vi "CO Serial CAL & Data Recording & DECADEv3.3.vi"() -> ()   [LabVIEW 2014]
uses:
  <vilib>/Platform/TimedLoop/XDataNode/timing_clust.ctl
  <vilib>/Platform/TimedLoop/XDataNode/nitl_modes.ctl
  <vilib>/Platform/TimedLoop/XDataNode/wakeup.ctl
  C:/Program Files (x86)/National Instruments/LabVIEW 2014/examples/Data Communication/Network Streams/Simple Network Streams/support/Network Stream Command.ctl
  <vilib>/Utility/error.llb/whitespace.ctl
  <vilib>/Instr/_visa.llb/VISA Configure Serial Port (Instr).vi
  <vilib>/Utility/tcp.llb/UDP Multicast Write-Only Open.vi
  <vilib>/platform/TimedLoop/XDataNode/XDataNode.xnode
  <vilib>/Platform/TimedLoop/XDataNode/XDNodeRunTimeDep.lvlib
panel:
  out "Stop File Write":bool
  out "Default file name":string
  in  "Flight Number 2":string="XXXX"
  out "status":bool
  out "CO Vacuum":bool
  out "CO CAL":bool
  out "error out":errorcluster
  out "CO Vacuum?":i16
  out "Control data":i32[](array[numeric])
  out "Control data out":string
  in  "VISA resource name":refnum<visa-resource-name>="ASRL8::INSTR"
  out "Serial VISA error":errorcluster
  out "SEPTIC TCP Error Out":errorcluster
  out "TCP packet\nSend To SEPTIC":bool
  in  "msec to wait":u32=330 caption="mSec to Wait"
  out "UDP Time Stamp Offset":i32=1
  out "Scan from String Error \nCounter from process loop":i32
  out "TCP Binary Packet":string
  in  "ue9LJ temp":u16
  out "FISH TCP Error Out":errorcluster
  out "TCP packet\nSend To FISH":bool
  out "UDP_Out_Error Out":errorcluster
  out "Data Array":string[](array[string])
  out "UDP_Out Status":bool
  out "Data Process Status":bool
  out "Command In":string[](array[string])
  out "ERR Counter":i32
  out "UDP_Out":string
  out "UDP_Pack_num":u32
  out "Flight Number":string
  out "OK RAW COUNTER":i32
  out "IN_CAL?":bool
  out "Redundent DATA":string
  out "Data String":string
  out "CO_Data_Buffer":string[](array[string])
  out "RAW DATA":string
  out "loop count":i32
  out "Number of Read error":i32
  out "Command In":string
  # "Pre-flight"
  # "CONC"
  # "SIG"
  # "SENS"
  # "ZERO"
  # "Lamp flow controller"
  # "Lamp temperature"
  # "Monochromater flow controller"
  # "Monochromater temperature"
  # "Monochromater pressure"
  # "Fluorescence cell pressure"
  # "Calibration gas pressure"
  # "Cell temperature"
  # "Calibration Concentration"
  # "ERROR number"
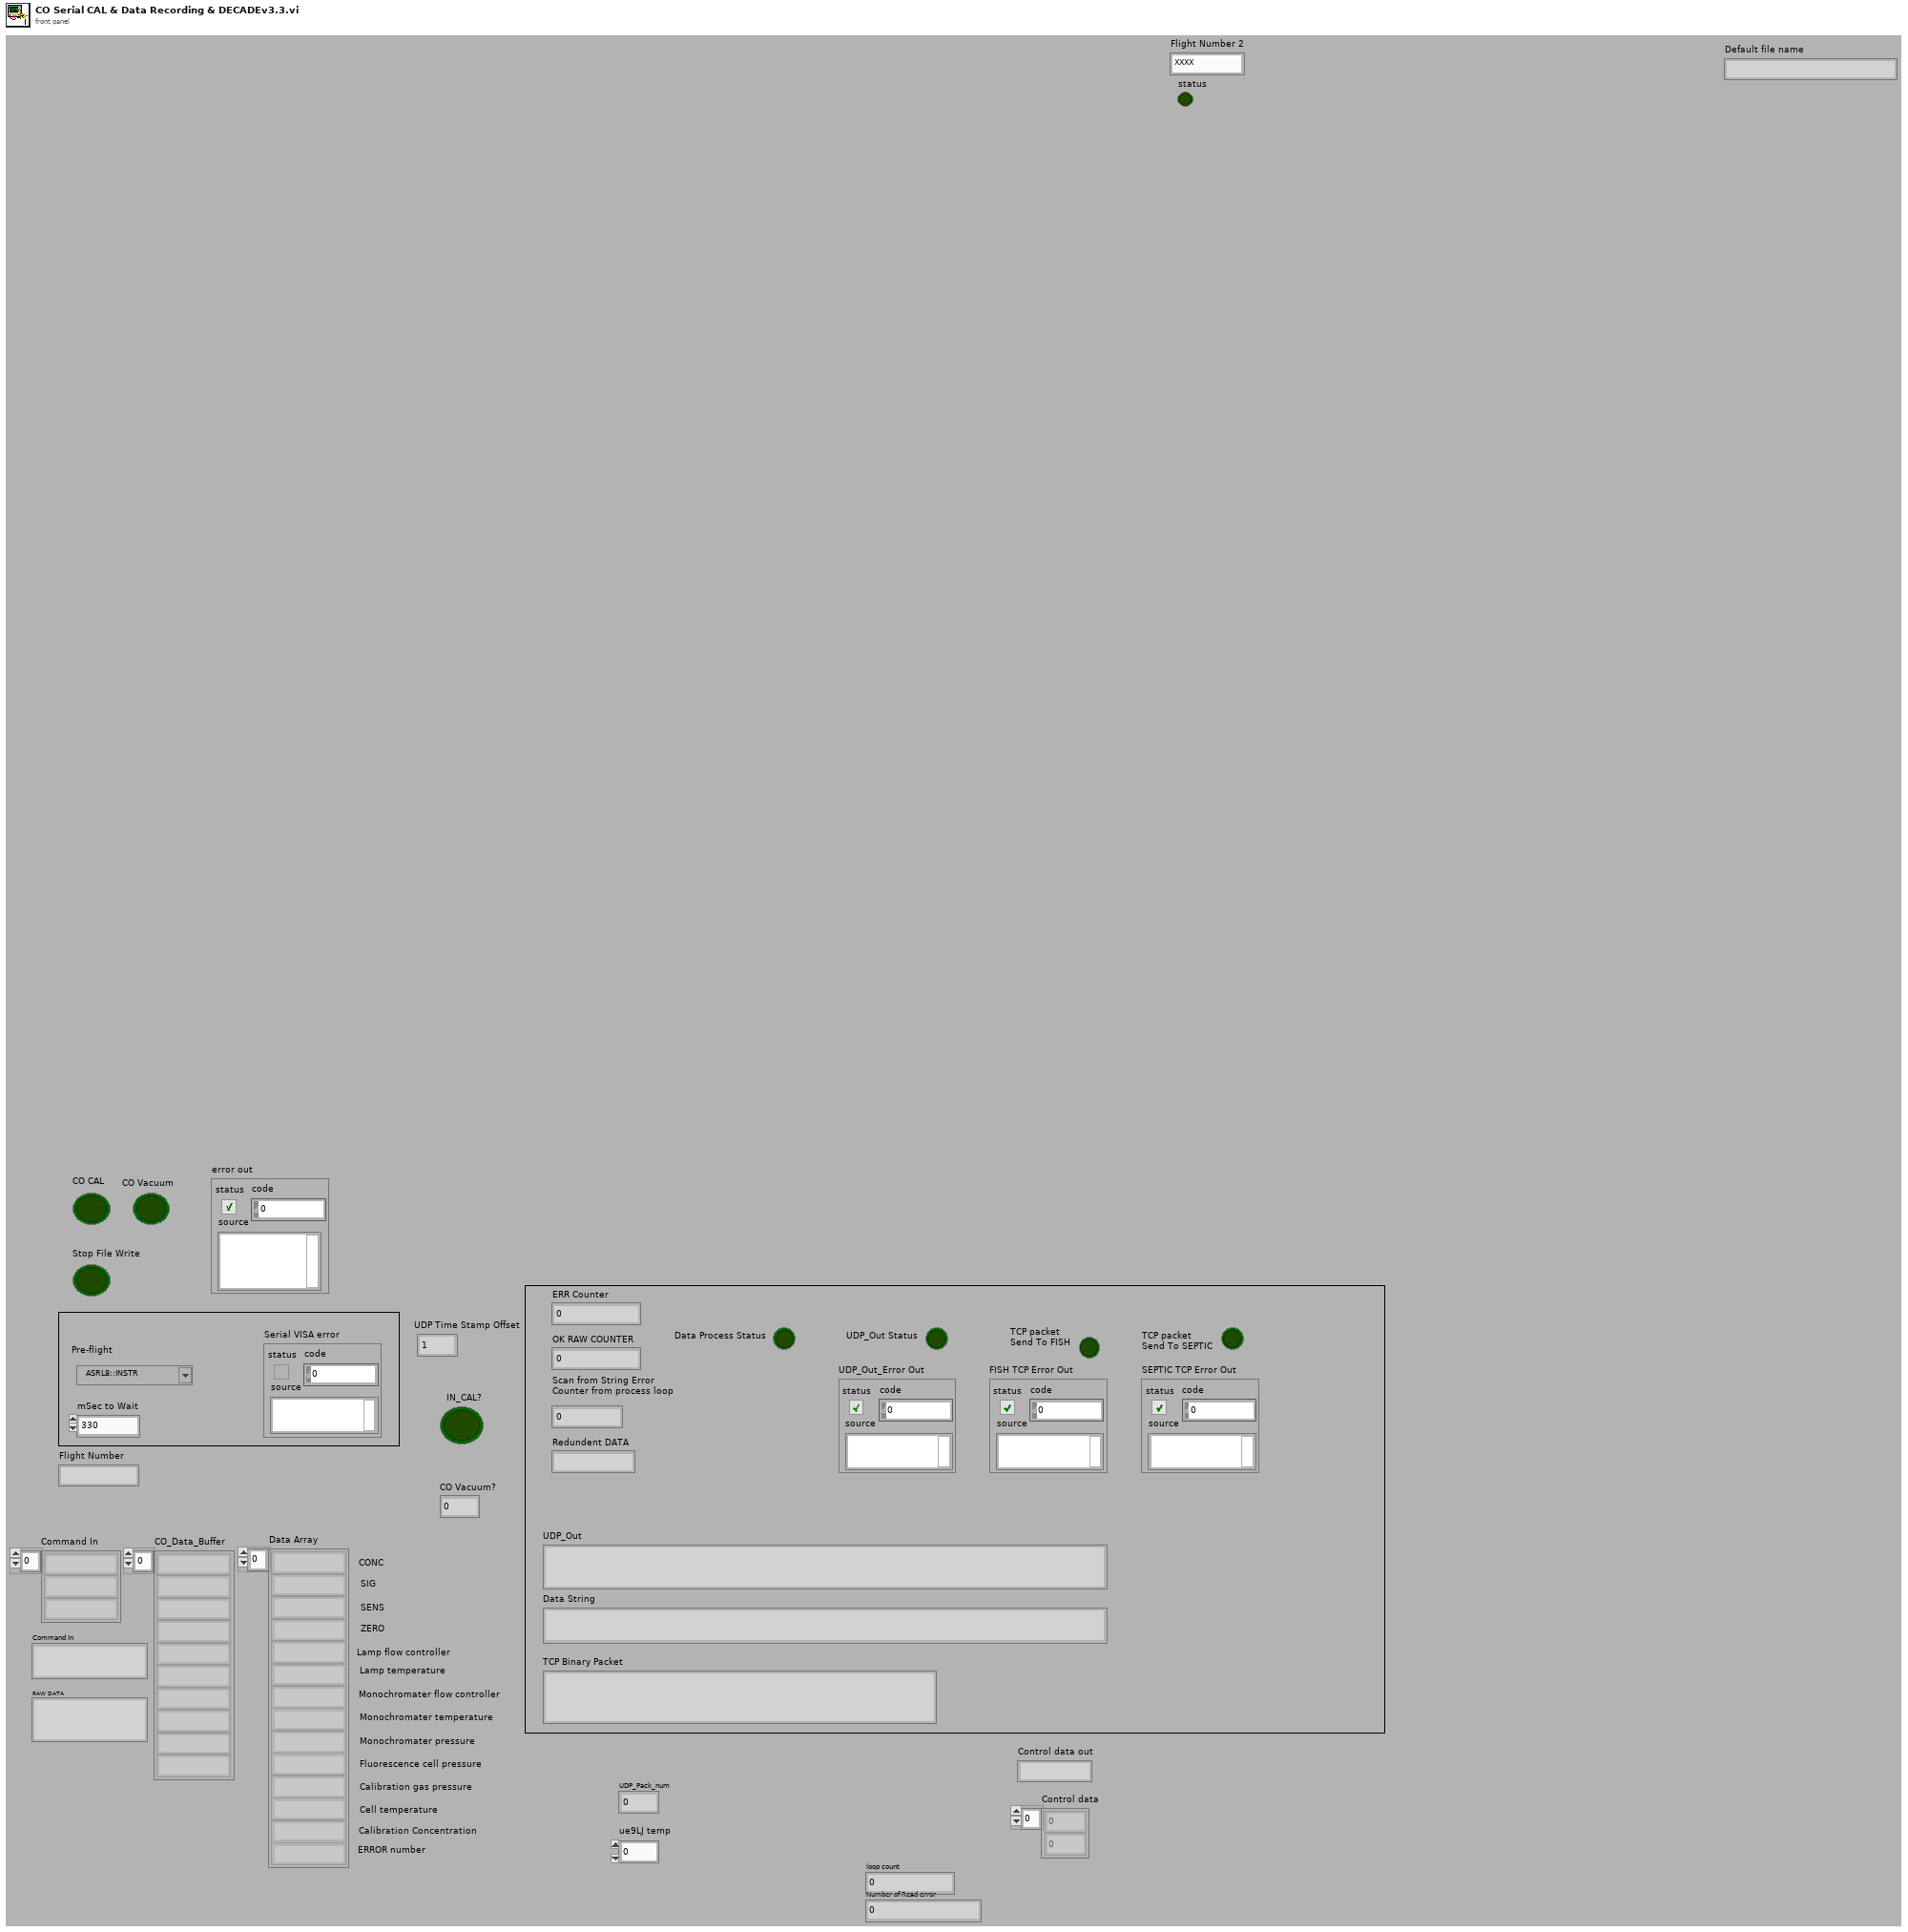
[diagram p1: front panel]
types:
  T1 = typedef "XDNodeRunTimeDep.lvlib/timing_clust.ctl" = cluster{"Expected End [f-1]":u64, "Actual End [f-1]":u64, "Finished Late? [f-1]":bool, "Expected End [i-1]":u64, "Actual End [i-1]":u64, "Finished Late? [i-1]":bool, "Expected Start [i]":u64, "Actual Start [i]":u64, "Expected Start [f]":u64, "Actual Start [f]":u64, "Source Name":string, "Structure Name":string, "Period":i64, "Deadline":i64, "Offset":i64, "Start":i64, "Priority":i32, "Timeout":i32, "Mode":T2, "Wakeup Reason":T3, "Error":errorcluster, "Source Type":string, "Secondary Source Type":string, "Global End Time":u64, "Global Start Time":u64, "Frame Duration":u64, "Iteration Duration":u64, "Assigned CPU":i32, "I/O Scan Engine Mode":u32}
  T2 = typedef "XDNodeRunTimeDep.lvlib/nitl_modes.ctl" = enum32{"No Change", "Process missed periods, maintain original phase", "Discard missed periods, maintain original phase", "Process missed periods, ignore original phase", "Discard missed periods, ignore original phase"}
  T3 = typedef "XDNodeRunTimeDep.lvlib/wakeup.ctl" = enum32{"Normal", "Aborted", "Asynchronous wakeup", "Timing source error", "Timed loop error", "Timeout"}
  T4 = typedef "Network Stream Command.ctl" = cluster{"Message":string, "Message Data":variant}
  T5 = enum16{"open", "replace", "create", "open or create", "replace or create", "replace or create with confirmation"}
  T6 = typedef "whitespace.ctl" = u16
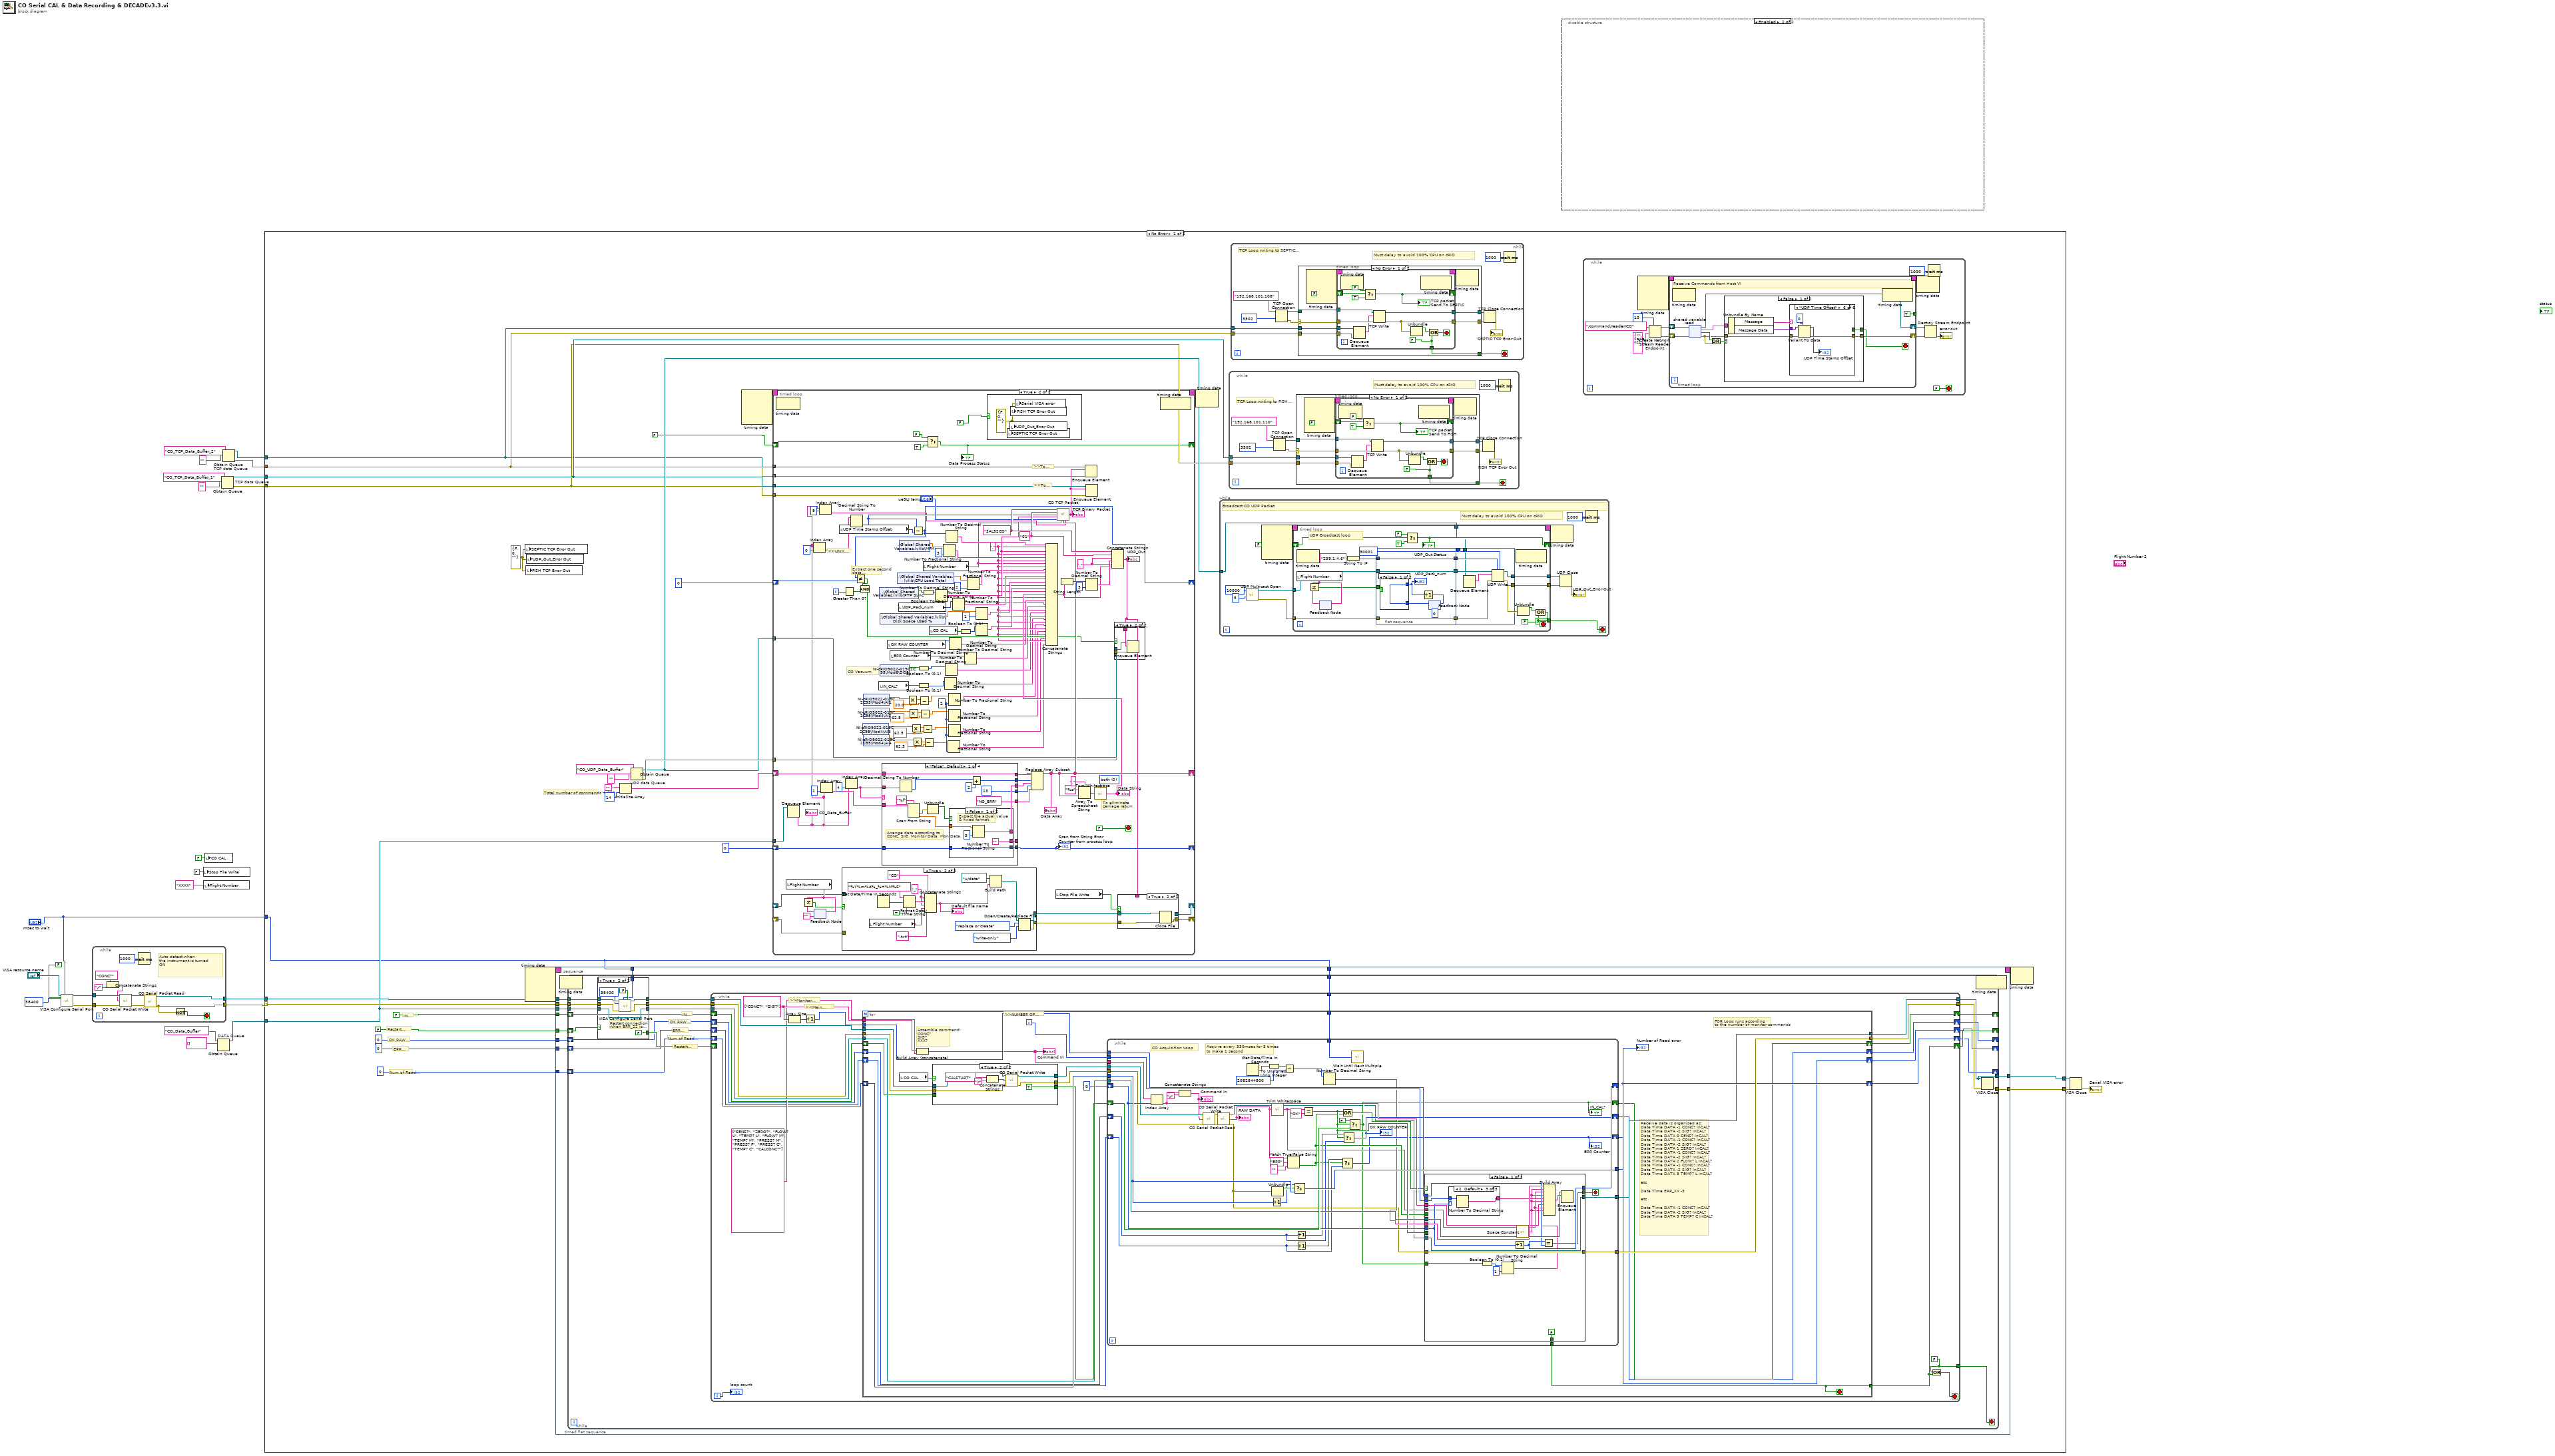
[diagram p0: block diagram]
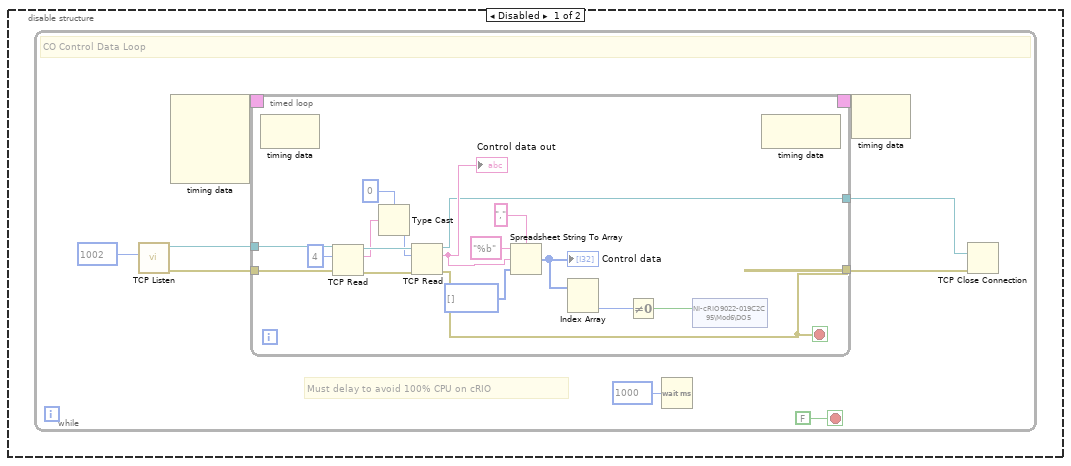
[diagram p2: hidden frame]
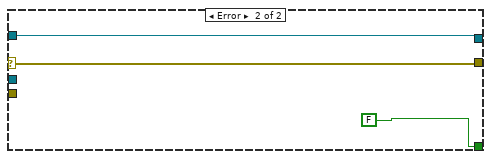
[diagram p3: hidden frame]
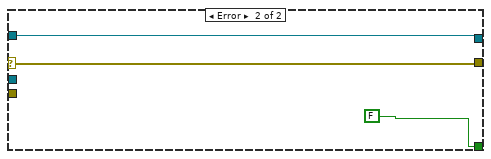
[diagram p4: hidden frame]
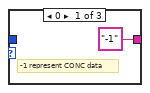
[diagram p6: hidden frame]
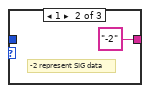
[diagram p7: hidden frame]
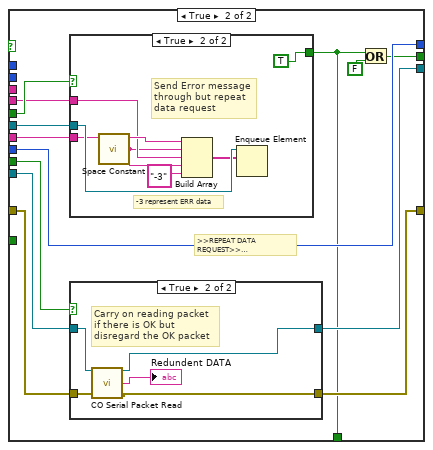
[diagram p8: hidden frame]
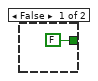
[diagram p10: hidden frame]
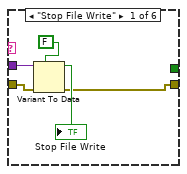
[diagram p12: hidden frame]
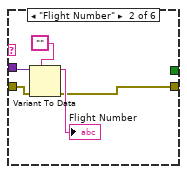
[diagram p13: hidden frame]
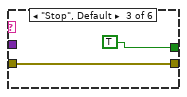
[diagram p14: hidden frame]
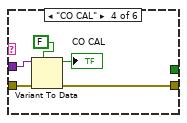
[diagram p15: hidden frame]
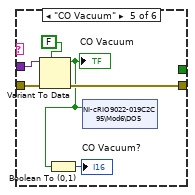
[diagram p16: hidden frame]
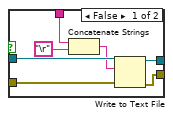
[diagram p19: hidden frame]
diagram:
  n1 = call-poly "VISA Configure Serial Port"("VISA resource name"="VISA resource name", "timeout (10sec)"="msec to wait", "Enable Termination\nChar (T)"=FALSE ("Enable Termination\nChar (T)"), "baud rate (9600)"=u32 38400) -> ("VISA resource name out"=w12:refnum<visa-resource-name>, "error out"=w11:errorcluster)  [unwired: 10 in]
  n2 = while {
    tunnel: w12 -> [w36]
    tunnel: w11 -> [w35]
    tunnel: [w29] -> w10
    tunnel: [w30] -> w9
    stop <- w34 stop-if-true
    # "Auto detect when\nthe instrument is turned \nON"
    n3 = Concatenate Strings("CONC?" ("Data in"), "\r") -> (w26:string)
    n4 = call "CO Serial Packet Write.vi"("VISA resource name In"=w36, "Data in"=w26, "error in (no error)"=w35) -> ("VISA resource name Out"=w32:refnum<visa-resource-name>, "error out"=w31:errorcluster)  [unwired: 11 in]
    n5 = Wait (ms)(milliseconds to wait=u32 1000) -> ()  [unwired: 1 out]
    n6 = call "CO Serial Packet Read.vi"("VISA resource In"=w32, "error in"=w31) -> ("VISA resource Out"=w29:refnum<visa-resource-name>, "error out"=w30:errorcluster)  [unwired: 11 in, 1 out]
    n7 = Not(x=w30) -> (.not. x?=w34:bool)
  }
  n8 = local write "Stop File Write"(FALSE ("Stop File Write")) -> ()
  n9 = local write "Flight Number"("XXXX" ("Flight Number")) -> ()
  n10 = local write "CO CAL"(FALSE ("CO CAL")) -> ()
  n11 = Obtain Queue "DATA Queue"(name (unnamed)="CO_Data_Buffer", element data type=string[] []) -> (queue out=w23:refnum<queue>)  [unwired: 3 in, 2 out]
  n12 = Obtain Queue "TCP data Queue"(name (unnamed)="CO_TCP_Data_Buffer_1", element data type="") -> (queue out=w22:refnum<queue>, error out=w21:errorcluster)  [unwired: 3 in, 1 out]
  n13 = Obtain Queue "TCP data Queue"(name (unnamed)="CO_TCP_Data_Buffer_2", element data type="") -> (queue out=w20:refnum<queue>, error out=w19:errorcluster)  [unwired: 3 in, 1 out]
  n14 = case shown="No Error" w9 {
    selector: w9 -> [w64 w714]
    tunnel: w10 -> [w65 w713]
    tunnel: [w66 w714] -> w15
    tunnel: [w42 w713] -> w14
    tunnel: w23 -> [w63 _]
    tunnel: w22 -> [w52 _]
    tunnel: w21 -> [w51 _]
    tunnel: w20 -> [w50 _]
    tunnel: w19 -> [w49 _]
    tunnel: "msec to wait" -> [w37 _]
    frame No Error {
      w48 = errorcluster {"status"=FALSE, "code"=0, "source"=""} ("UDP_Out_Error Out")
      # "Restart connection?"
      # "IN CAL?"
      # "OK RAW Counter"
      # "ERR Counter"
      # "Num of Read Error"
      # "Total number of commands + ERR"
      n15 = node-c288() -> (w39:T1)  [unwired: 4 in]
      n16 = local write "SEPTIC TCP Error Out"(w48) -> ()
      n17 = local write "FISH TCP Error Out"(w48) -> ()
      n18 = local write "UDP_Out_Error Out"(w48) -> ()
      n19 = timed-sequence {
        timing: w39 -> [_]
        timing-out: [_] -> w38
        tunnel: [w162] -> w66
        tunnel: w65 -> [w161]
        tunnel: w64 -> [w160]
        tunnel: w63 -> [w159]
        tunnel: FALSE -> [w158]
        tunnel: 0 -> [w157]
        tunnel: 0 -> [w156]
        tunnel: 0 -> [w155]
        tunnel: FALSE ("IN_CAL?") -> [w154]
        tunnel: [w153] -> w42
        tunnel: w37 -> [w152]
        tunnel: w37 -> [w151]
        n20 = timed-flat-sequence {
          tunnel: [w174] -> w162
          tunnel: w161 -> [w173]
          tunnel: w160 -> [w172]
          tunnel: w159 -> [w171]
          tunnel: w158 -> [w170]
          tunnel: w157 -> [w169]
          tunnel: w156 -> [w168]
          tunnel: w155 -> [w167]
          tunnel: w154 -> [w166]
          tunnel: [w165] -> w153
          tunnel: w152 -> [w164]
          tunnel: w151 -> [w163]
          n21 = node-c288() -> ()  [unwired: 1 in, 1 out]
          n22 = while {
            tunnel: [w179] -> w174
            tunnel: w173 -> [w196]
            tunnel: w172 -> [w195]
            tunnel: w171 -> [w193]
            shift-right: [w190] -> _
            shift-left: w170 -> [w191]
            shift-right: [w186] -> _
            shift-left: w169 -> [w187]
            shift-right: [w183] -> _
            shift-left: w168 -> [w185]
            shift-right: [w182] -> _
            shift-left: w167 -> [w184]
            shift-right: [w180] -> _
            shift-left: w166 -> [w181]
            tunnel: [w177] -> w165
            tunnel: w164 -> [w176]
            tunnel: w163 -> [w175]
            stop <- w189 stop-if-true
            # "Restart connection?"
            # "Num of Read Error"
            # "ERR Counter"
            # "IN CAL?"
            # "OK RAW Counter"
            n23 = case shown="True" w191 {
              selector: w191 -> [w198 _]
              tunnel: [w201 w207] -> w197
              tunnel: w196 -> [w201 w208]
              tunnel: [w200 w206] -> w194
              tunnel: w195 -> [w200 w205]
              tunnel: [w199 w210] -> w192
              tunnel: w193 -> [w199 w210]
              tunnel: [w198 FALSE] -> w188
              tunnel: w175 -> [_ w202]
              frame False {
              }
              frame True {
                # "Restart connection\nwhen ERR_22 is detected"
                n24 = call-poly "VISA Configure Serial Port"("VISA resource name"=w208, "timeout (10sec)"=w202, "Enable Termination\nChar (T)"=FALSE ("Enable Termination\nChar (T)"), "baud rate (9600)"=u32 38400, "error in (no error)"=w205) -> ("VISA resource name out"=w207:refnum<visa-resource-name>, "error out"=w206:errorcluster)  [unwired: 9 in]
              }
            }
            n25 = while {
              tunnel: [w232] -> w178
              tunnel: w197 -> [w231]
              tunnel: w194 -> [w230]
              tunnel: [w229] -> w177
              tunnel: w192 -> [w228]
              shift-right: [w219] -> w186
              shift-left: w187 -> [w223]
              shift-right: [w218] -> w183
              shift-left: w185 -> [w222]
              shift-right: [w217] -> w180
              shift-left: w181 -> [w221]
              shift-right: [w216] -> w182
              shift-left: w184 -> [w220]
              tunnel: [w212] -> w189
              shift-right: [w213] -> w190
              shift-left: w188 -> [_]
              tunnel: w176 -> [w211]
              i -> [w215]
              stop <- w214 stop-if-true
              w212 = FALSE
              w227 = string[] ["CONC?", "SIG?"]
              # ">>Main commands>>"
              # ">>Monitor Command>>"
              n26 = Array Size(array=w227) -> (size(s)=w224:i32)
              n27 = Increment(x=w224) -> (x+1=w226:i32)
              n28 = for {
                tunnel: w231 -> [w252]
                tunnel: w230 -> [w251]
                tunnel: [w257] -> w232
                shift-right: [w255] -> w216
                shift-left: w220 -> [w256]
                tunnel: [w254] -> w229
                tunnel: w228 -> [w253]
                tunnel: w226 -> [w247]
                shift-right: [w245] -> w217
                shift-left: w221 -> [w246]
                shift-right: [w243] -> w218
                shift-left: w222 -> [w244]
                shift-right: [w241] -> w219
                shift-left: w223 -> [w242]
                tunnel: string[] ["SENS?", "ZERO?", "FLOW? L", "TEMP? L", "FLOW? M", "TEMP? M", "PRESS? M", "PRESS? F", "PRESS? C", "TEMP? C", "CALCONC?"] -> [w238] mode=indexing
                tunnel: w227 -> [w239]
                tunnel: [w236] -> w213
                tunnel: w211 -> [w234]
                i -> [w237]
                stop <- w236 stop-if-true
                # "Receive data is organised as:\nDate Time DATA -1 CONC? InCAL?\nDate Time DATA -2 SIG? InCAL?\nDate Time DATA 0 SENS? InCAL?\nDate Time DATA -1 CONC? InCAL?\nDate Time DATA -2 SIG? InCAL?\nDate Time DATA 1 ZERO? InCAL?\nDate Time DATA -1 CONC? InCAL?\nDate Time DATA -2 SIG? InCAL?\nDate Time DATA 2 FLOW? L InCAL?\nDate Time DATA -1 CONC? InCAL?\nDate Time DATA -2 SIG? InCAL?\nDate Time DATA 3 TEMP? L InCAL?\n\netc\n\nDate Time ERR_XX -3\n\netc\n\nDate Time DATA -1 CONC? InCAL?\nDate Time DATA -2 SIG? InCAL?\nDate Time DATA 9 TEMP? C InCAL?"
                # "FOR Loop runs according\nto the number of monitor commands"
                # "Assemble command:\nCONC?\nSIG?\nXXX?"
                # ">>NUMBER OF COMMANDS>>"
                n29 = local read "CO CAL"() -> (w233:bool)
                n30 = Build Array (concatenate)(w239, w238) -> (w240:string[])
                "Command In" <- w240
                n31 = case shown="True" w233 {
                  tunnel: w252 -> [w357 w359]
                  tunnel: w251 -> [w356 w362]
                  tunnel: [w357 w360] -> w250
                  tunnel: [w356 w361] -> w249
                  tunnel: [w355 TRUE ("IN_CAL?")] -> w248
                  tunnel: w246 -> [w355 _]
                  frame False {
                  }
                  frame True {
                    n32 = Concatenate Strings("CALSTART" ("string"), "\r") -> (w358:string)
                    n33 = call "CO Serial Packet Write.vi"("VISA resource name In"=w359, "Data in"=w358, "error in (no error)"=w362) -> ("VISA resource name Out"=w360:refnum<visa-resource-name>, "error out"=w361:errorcluster)  [unwired: 11 in]
                  }
                }
                n34 = while {
                  tunnel: w249 -> [w264]
                  tunnel: [w291] -> w257
                  tunnel: w256 -> [w303]
                  tunnel: [w302] -> w255
                  tunnel: w240 -> [w295]
                  tunnel: [w292] -> w254
                  tunnel: w253 -> [w290]
                  tunnel: w250 -> [w266]
                  shift-right: [w267] -> w245
                  shift-left: w248 -> [w297]
                  shift-right: [w294] -> _
                  shift-left: 0 -> [w296]
                  tunnel: w247 -> [w287]
                  shift-right: [w284] -> w243
                  shift-left: w244 -> [w285]
                  shift-right: [w278] -> w241
                  shift-left: w242 -> [w280]
                  tunnel: w237 -> [w277]
                  tunnel: [w272] -> w236
                  tunnel: w234 -> [w258]
                  stop <- w293 stop-if-true
                  # "Acquire every 330msec for 3 times\nto make 1 second"
                  # "CO Acquisition Loop"
                  n35 = Index Array(array=w295, index=w296) -> (element=w289:string)
                  n36 = Concatenate Strings(w289, "\r") -> (w265:string)
                  "Command In" <- w265
                  n37 = call "CO Serial Packet Write.vi"("VISA resource name In"=w266, "Data in"=w265, "error in (no error)"=w264) -> ("VISA resource name Out"=w262:refnum<visa-resource-name>, "error out"=w263:errorcluster)  [unwired: 11 in]
                  n38 = call "CO Serial Packet Read.vi"("VISA resource In"=w262, "error in"=w263) -> ("VISA resource Out"=w261:refnum<visa-resource-name>, "Data Out"=w259:string, "error out"=w260:errorcluster)  [unwired: 11 in]
                  "RAW DATA" <- w259
                  n39 = Get Date/Time In Seconds() -> (seconds since 1Jan1904=w273:timestamp)
                  n40 = To Unsigned Long Integer(number=w273) -> (unsigned 32bit integer=w276:u32)
                  n41 = Increment(x=w303) -> (x+1=w299:i32)
                  n42 = call <vilib>:"Trim Whitespace.vi"("string"=w259) -> ("trimmed string"=w271:string)  [unwired: 1 in]
                  n43 = Unbundle(w260) -> ("status"=w300:bool)  [unwired: 2 out]
                  n44 = Subtract(x=w276, y=u32 2082844800) -> (x-y=w268:u32)
                  n45 = Match True/False String(2:"" ("false string"), 3:"ERR" ("true string"), 4:w259) -> (0:w279:bool)  [unwired: 1 out]
                  n46 = Select(t=w299, s=w300, f=w303) -> (s? t:f=w302:i32)
                  n47 = Increment(x=w285) -> (x+1=w286:i32)
                  n48 = Increment(x=w280) -> (x+1=w281:i32)
                  n49 = Equal?(x=w271, y="OK" ("string")) -> (x = y?=w282:bool)
                  n50 = Number To Decimal String(number=w268) -> (decimal integer string=w274:string)  [unwired: 1 in]
                  n51 = Select(t=w281, s=w279, f=w280) -> (s? t:f=w278:i32)
                  "ERR Counter" <- w278
                  n52 = Select(t=w286, s=w282, f=w285) -> (s? t:f=w284:i32)
                  "OK RAW COUNTER" <- w284
                  n53 = Compound Arithmetic op=OR(w282, w279) -> (w283:bool)
                  n54 = Select(t=FALSE, s=w282, f=w297) -> (s? t:f=w267:bool)
                  "IN_CAL?" <- w267
                  n55 = call "Wait Until Next Multiple"("Count(mSec)"=w258) -> ()  [unwired: 1 out]
                  n56 = case shown="False" w283 {
                    tunnel: w296 -> [w311 w339]
                    tunnel: [w322 w339] -> w294
                    tunnel: [w316 w329] -> w293
                    tunnel: w261 -> [w321 w338]
                    tunnel: w260 -> [w320 w337]
                    tunnel: [w321 w336] -> w292
                    tunnel: [w320 w335] -> w291
                    tunnel: w290 -> [w318 w333]
                    tunnel: w271 -> [w309 w331]
                    tunnel: w289 -> [w312 _]
                    tunnel: w274 -> [w317 w332]
                    tunnel: w279 -> [_ w334]
                    tunnel: w287 -> [w315 _]
                    tunnel: w282 -> [_ w330]
                    tunnel: w277 -> [w314 _]
                    tunnel: [FALSE w327] -> w272
                    tunnel: w267 -> [w308 _]
                    frame False {
                      n57 = case shown="2, Default" w311 {
                        tunnel: w314 -> [_ _ w326]
                        tunnel: ["-1" "-2" w325] -> w313
                        frame 0 {
                          # "-1 represent CONC data"
                        }
                        frame 1 {
                          # "-2 represent SIG data"
                        }
                        frame 2, Default {
                          n58 = Number To Decimal String(number=w326) -> (decimal integer string=w325:string)  [unwired: 1 in]
                        }
                      }
                      n59 = Boolean To (0,1)(Boolean=w308) -> (0, 1=w307:i16)
                      n60 = Number To Decimal String(number=w307, width (-)=i16 1) -> (decimal integer string=w304:string)
                      n61 = Increment(x=w311) -> (x+1=w322:i32)
                      n62 = call <vilib>:"Space Constant.vi"() -> ("String"=w305:string)
                      n63 = Equal?(x=w322, y=w315) -> (x = y?=w316:bool)
                      n64 = Build Array(w317, w305, w309, w305, w313, w305, w312, w309, w305, w304) -> (w319:string[])
                      n65 = Enqueue Element(queue=w318, element=w319) -> ()  [unwired: 2 in, 3 out]
                    }
                    frame True {
                      # ">>REPEAT DATA REQUEST>>\nif OK or ERR"
                      n66 = case shown="True" w334 {
                        tunnel: w333 -> [_ w354]
                        tunnel: w332 -> [_ w352]
                        tunnel: w331 -> [_ w351]
                        tunnel: [FALSE TRUE] -> w327
                        frame False {
                        }
                        frame True {
                          # "-3 represent ERR data"
                          # "Send Error message\nthrough but repeat\ndata request"
                          n67 = call <vilib>:"Space Constant.vi"() -> ("String"=w350:string)
                          n68 = Build Array(w352, w350, w351, w350, "-3" ("element")) -> (w353:string[])
                          n69 = Enqueue Element(queue=w354, element=w353) -> ()  [unwired: 2 in, 3 out]
                        }
                      }
                      n70 = case shown="True" w330 {
                        tunnel: w338 -> [w340 w345]
                        tunnel: w337 -> [w341 w346]
                        tunnel: [w340 w344] -> w336
                        tunnel: [w341 w342] -> w335
                        frame False {
                        }
                        frame True {
                          # "Carry on reading packet\nif there is OK but\ndisregard the OK packet"
                          n71 = call "CO Serial Packet Read.vi"("VISA resource In"=w345, "error in"=w346) -> ("VISA resource Out"=w344:refnum<visa-resource-name>, "Data Out"=→"Redundent DATA":string, "error out"=w342:errorcluster)  [unwired: 11 in]
                        }
                      }
                      n72 = Or(x=w327, y=FALSE) -> (x .or. y?=w329:bool)
                    }
                  }
                }
                "Number of Read error" <- w255
              }
              n73 = Or(x=w212, y=w213) -> (x .or. y?=w214:bool)
              "loop count" <- w215
            }
            n74 = VISA Close(VISA resource name=w177, error in (no error)=w178) -> (error out=w179:errorcluster)
          }
          n75 = node-c288() -> ()  [unwired: 1 in, 1 out]
        }
      }
      n76 = Initialize Array("", 14) -> (w60:string[])
      n77 = Obtain Queue "UDP data Queue"(name (unnamed)="CO_UDP_Data_Buffer", element data type="") -> (queue out=w55:refnum<queue>, error out=w56:errorcluster)  [unwired: 3 in, 1 out]
      n78 = node-c288() -> (w41:T1)  [unwired: 4 in]
      n79 = timed-loop {
        tunnel: w63 -> [w547]
        shift-right: [w518] -> _
        shift-left: w60 -> [w535]
        shift-right: [w522] -> _
        shift-left: FALSE -> [w525]
        tunnel: w52 -> [w517]
        tunnel: w51 -> [w516]
        tunnel: w55 -> [w514]
        tunnel: w56 -> [w513]
        shift-right: [w511] -> _
        shift-left: 0 -> [w512]
        shift-right: [w498] -> _
        shift-left: 0 -> [w505]
        tunnel: w50 -> [w503]
        tunnel: w49 -> [w502]
        timing: w41 -> [_]
        timing-out: [_] -> w40
        shift-right: [w487] -> _
        shift-left: _ -> [w480]
        shift-right: [w478] -> _
        shift-left: _ -> [w479]
        i -> [w508]
        stop <- FALSE stop-if-true
        w461 = 62.5 ("y")
        w462 = 62.5 ("y")
        w465 = 62.5 ("y")
        w468 = 20.0 ("y")
        w491 = i16 2 ("precision (6)")
        w527 = T6 0 items=["both", "start of string", "end of string"] ("location (both)")
        w443 = ","
        w520 = "01"
        w538 = ","
        w521 = "$AL52CO"
        # "CO Vacuum"
        # ">>To SEPTIC>>"
        # ">>To FISH>>"
        # "Extract one second data\nfor UDP sending"
        # ">>UNIX TIME>>"
        # "To eliminate\ncarriage return"
        n80 = node-c288() -> ()  [unwired: 1 in, 1 out]
        n81 = local read "Flight Number"() -> (w485:string)
        n82 = Dequeue Element(queue=w547) -> (element=w494:string[])  [unwired: 2 in, 3 out]
        "CO_Data_Buffer" <- w494
        n83 = Index Array(array=w494, index=0) -> (element=w506:string)
        n84 = feedback #1("" ("Flight Number")) -> (w484:string)
        n85 = Not Equal?(x=w485, y=w484) -> (x != y?=w483:bool)
        n86 = feedback-in #1(w485) -> ()
        n87 = Index Array(array=w494, index=9) -> (element=w493:string)
        n88 = Index Array(array=w494, index=2) -> (element=w533:string)
        n89 = local read "UDP Time Stamp Offset"() -> (w432:i32)
        n90 = case shown="True" w483 {
          tunnel: [w549 w551] -> w482
          tunnel: [w548 w550] -> w481
          tunnel: w480 -> [w549 _]
          tunnel: w479 -> [w548 _]
          frame False {
          }
          frame True {
            w558 = "_" ("string")
            n91 = local read "Flight Number"() -> (w564:string)
            n92 = Get Date/Time In Seconds() -> (seconds since 1Jan1904=w559:timestamp)
            n93 = Format Date/Time String(time format string (%c)="%Y%m%d%_%H%M%S", seconds (now)=w559, UTC format=TRUE) -> (date/time string=w562:string)
            n94 = Concatenate Strings("CO" ("string"), w558, w562, w558, w564, ".txt" ("string")) -> (w556:string)
            "Default file name" <- w556
            n95 = Build Path(base path=path "u:/data", name or relative path=w556) -> (appended path=w552:path)
            n96 = Open/Create/Replace File(file path (use dialog)=w552, operation (0:open)=T5."replace or create", access (0:read/write)=enum16{"read/write", "read-only", "write-only"}."write-only") -> (refnum out=w551:refnum<file>, error out=w550:errorcluster)  [unwired: 3 in, 1 out]
          }
        }
        n97 = Greater Than 0?(x=w508) -> (x > 0?=w507:bool)
        n98 = Index Array(array=w494, index=4) -> (element=w534:string)
        n99 = Decimal String To Number(string=w506) -> (number=w500:i32)  [unwired: 2 in, 1 out]
        n100 = shared-variable "NI-cRIO9022-019C2C95\\Mod4\\AI3"() -> (w460:dbl)  [unwired: 1 in, 1 out]
        n101 = shared-variable "NI-cRIO9022-019C2C95\\Mod4\\AI4"() -> (w458:dbl)  [unwired: 1 in, 1 out]
        n102 = shared-variable "NI-cRIO9022-019C2C95\\Mod4\\AI1"() -> (w470:dbl)  [unwired: 1 in, 1 out]
        n103 = shared-variable "NI-cRIO9022-019C2C95\\Mod4\\AI2"() -> (w464:dbl)  [unwired: 1 in, 1 out]
        n104 = local read "IN_CAL?"() -> (w442:bool)
        n105 = shared-variable ".\\Global Shared Variables.lvlib\\PTP Sync"() -> (w471:bool)  [unwired: 1 in, 1 out]
        n106 = shared-variable ".\\Global Shared Variables.lvlib\\Disk Space Used %"() -> (w448:dbl)  [unwired: 1 in, 1 out]
        n107 = shared-variable "NI-cRIO9022-019C2C95\\Mod6\\DO5"() -> (w434:bool)  [unwired: 1 in, 1 out]
        n108 = case shown="\"False\", Default" w534 {
          tunnel: w534 -> [w595 _ _ _]
          tunnel: w535 -> [w596 w618 w640 w654]
          tunnel: w533 -> [w587 w612 w634 w650]
          tunnel: [w596 w618 w640 w654] -> w532
          tunnel: [w593 0 ("index") 1 ("index") w651] -> w531
          tunnel: [w586 w608 w630 w650] -> w530
          tunnel: [w585 w609 w631 ""] -> _
          tunnel: w512 -> [w584 w611 w633 w652]
          tunnel: [w583 w610 w632 w652] -> w511
          tunnel: [13 ("index") 13 ("index") 13 ("index") w651] -> w497
          tunnel: ["NO_ERR" "NO_ERR" "NO_ERR" w650] -> w496
          frame "False", Default {
            # "Arrange data according to\nCONC, SIG, Monitor Data, Mon Data,"
            n109 = Decimal String To Number(string=w595) -> (number=w592:i32)  [unwired: 2 in, 1 out]
            n110 = Scan From String(format string="%f", input string=w587) -> (error out=w589:errorcluster, output 1=w590:dbl)  [unwired: 3 in, 2 out]
            n111 = Unbundle(w589) -> ("status"=w588:bool)  [unwired: 2 out]
            n112 = case shown="False" w588 {
              tunnel: [w601 ""] -> w586
              tunnel: w590 -> [w600 _]
              tunnel: w584 -> [w599 w604]
              tunnel: [w599 w603] -> w583
              tunnel: ["" "Scan from string error"] -> w585
              frame False {
                # "Extract the actual value\n& fixed format"
                n113 = Number To Fractional String(number=w600, precision (6)=i16 3) -> (F-format string=w601:string)  [unwired: 2 in]
              }
              frame True {
                # "If scan from string error,\nreplace data with empty\nstring"
                n114 = Increment(x=w604) -> (x+1=w603:i32)
              }
            }
            n115 = Add(x=w592, y=2) -> (x+y=w593:i32)
          }
          frame "-1" {
            # "Arrange data according to\nCONC, SIG, Monitor Data, Mon Data,"
            # "-1 represent CONC data"
            n116 = Scan From String(format string="%f", input string=w612) -> (error out=w614:errorcluster, output 1=w615:dbl)  [unwired: 3 in, 2 out]
            n117 = Unbundle(w614) -> ("status"=w613:bool)  [unwired: 2 out]
            n118 = case shown="False" w613 {
              tunnel: [w623 ""] -> w608
              tunnel: w615 -> [w622 _]
              tunnel: w611 -> [w621 w626]
              tunnel: [w621 w625] -> w610
              tunnel: ["" "Scan from string error"] -> w609
              frame False {
                # "Extract the actual value\n& fixed format"
                n119 = Number To Fractional String(number=w622, precision (6)=i16 5) -> (F-format string=w623:string)  [unwired: 2 in]
              }
              frame True {
                # "If scan from string error,\nreplace data with empty\nstring"
                n120 = Increment(x=w626) -> (x+1=w625:i32)
              }
            }
          }
          frame "-2" {
            # "Arrange data according to\nCONC, SIG, Monitor Data, Mon Data,"
            # "-2 represent SIG data"
            n121 = Scan From String(format string="%f", input string=w634) -> (error out=w636:errorcluster, output 1=w637:dbl)  [unwired: 3 in, 2 out]
            n122 = Unbundle(w636) -> ("status"=w635:bool)  [unwired: 2 out]
            n123 = case shown="False" w635 {
              tunnel: [w645 ""] -> w630
              tunnel: w637 -> [w644 _]
              tunnel: w633 -> [w643 w648]
              tunnel: [w643 w647] -> w632
              tunnel: ["" "Scan from string error"] -> w631
              frame False {
                # "Extract the actual value\n& fixed format"
                n124 = Number To Fractional String(number=w644, precision (6)=i16 3) -> (F-format string=w645:string)  [unwired: 2 in]
              }
              frame True {
                # "If scan from string error,\nreplace data with empty\nstring"
                n125 = Increment(x=w648) -> (x+1=w647:i32)
              }
            }
          }
          frame "-3" {
            w651 = 13 ("index")
            # "-3 represent ERR data"
          }
        }
        "Scan from String Error \nCounter from process loop" <- w511
        n126 = local read "OK RAW COUNTER"() -> (w536:i32)
        n127 = local read "ERR Counter"() -> (w490:i32)
        n128 = shared-variable ".\\Global Shared Variables.lvlib\\CPU Load Total"() -> (w476:dbl)  [unwired: 1 in, 1 out]
        n129 = local read "UDP_Pack_num"() -> (w543:u32)
        n130 = shared-variable ".\\Global Shared Variables.lvlib\\MFM"() -> (w475:dbl)  [unwired: 1 in, 1 out]
        n131 = Multiply(x=w470, y=w468) -> (x*y=w469:dbl)
        n132 = Multiply(x=w464, y=w465) -> (x*y=w466:dbl)
        n133 = Multiply(x=w460, y=w462) -> (x*y=w459:dbl)
        n134 = Multiply(x=w458, y=w461) -> (x*y=w457:dbl)
        n135 = Subtract(x=w500, y=w432) -> (x-y=w498:i32)
        n136 = Not Equal?(x=w498, y=w505) -> (x != y?=w509:bool)
        n137 = Compound Arithmetic op=AND(w509, w507) -> (w504:bool)
        n138 = Boolean To (0,1)(Boolean=w434) -> (0, 1=w433:i16)
        n139 = Boolean To (0,1)(Boolean=w442) -> (0, 1=w441:i16)
        n140 = Subtract(x=w469, y=w468) -> (x-y=w467:dbl)
        n141 = Subtract(x=w466, y=w465) -> (x-y=w463:dbl)
        n142 = Subtract(x=w459, y=w462) -> (x-y=w456:dbl)
        n143 = Boolean To (0,1)(Boolean=w471) -> (0, 1=w472:i16)
        n144 = local read "Flight Number"() -> (w452:string)
        n145 = Subtract(x=w457, y=w461) -> (x-y=w455:dbl)
        n146 = Select(t=FALSE, s=w525, f=TRUE) -> (s? t:f=w522:bool)
        "Data Process Status" <- w522
        n147 = local read "CO CAL"() -> (w446:bool)
        n148 = Number To Decimal String(number=w472) -> (decimal integer string=w454:string)  [unwired: 1 in]
        n149 = Number To Fractional String(number=w475, precision (6)=i16 3 ("width (-)")) -> (F-format string=w453:string)  [unwired: 2 in]
        n150 = Number To Decimal String(number=w441) -> (decimal integer string=w439:string)  [unwired: 1 in]
        n151 = Number To Decimal String(number=w433) -> (decimal integer string=w440:string)  [unwired: 1 in]
        n152 = Number To Decimal String(number=w498) -> (decimal integer string=w499:string)  [unwired: 1 in]
        n153 = Number To Fractional String(number=w455, precision (6)=w491) -> (F-format string=w435:string)  [unwired: 2 in]
        n154 = Number To Fractional String(number=w467, precision (6)=w491) -> (F-format string=w438:string)  [unwired: 2 in]
        n155 = Number To Fractional String(number=w463, precision (6)=w491) -> (F-format string=w437:string)  [unwired: 2 in]
        n156 = Number To Fractional String(number=w456, precision (6)=w491) -> (F-format string=w436:string)  [unwired: 2 in]
        n157 = Number To Decimal String(number=w536) -> (decimal integer string=w542:string)  [unwired: 1 in]
        n158 = Number To Decimal String(number=w543) -> (decimal integer string=w450:string)  [unwired: 1 in]
        n159 = Boolean To (0,1)(Boolean=w446) -> (0, 1=w447:i16)
        n160 = Number To Decimal String(number=w490) -> (decimal integer string=w489:string)  [unwired: 1 in]
        n161 = Number To Fractional String(number=w476, precision (6)=i16 2 ("width (-)")) -> (F-format string=w451:string)  [unwired: 2 in]
        n162 = Number To Fractional String(number=w448, precision (6)=i16 1 ("width (-)")) -> (F-format string=w445:string)  [unwired: 2 in]
        n163 = Number To Decimal String(number=w447) -> (decimal integer string=w444:string)  [unwired: 1 in]
        n164 = case shown="True" FALSE {
          frame False {
          }
          frame True {
            w577 = errorcluster {"status"=FALSE, "code"=0, "source"=""} ("UDP_Out_Error Out")
            n165 = local write "SEPTIC TCP Error Out"(w577) -> ()
            n166 = local write "UDP_Out_Error Out"(w577) -> ()
            n167 = local write "FISH TCP Error Out"(w577) -> ()
            n168 = local write "Serial VISA error"(w577) -> ()
          }
        }
        n169 = Replace Array Subset(array=w532, new element #1=w530, index #1=w531, new element #2=w496, index #2=w497) -> (w518:string[])
        "Data Array" <- w518
        n170 = local read "Stop File Write"() -> (w486:bool)
        n171 = call "CO TCP Packet.vi"("ID"=w521, "Version"=w520, "utc_time"=w500, "PTP Sync"=w454, "ue9LJ temp"="ue9LJ temp", "Flight Number"=w452, "Data Array"=w518, "In_CAL?"=w493) -> ("TCP Binary Packet"=w501:string)  [unwired: 7 in]
        "TCP Binary Packet" <- w501
        n172 = Array To Spreadsheet String(delimiter (Tab)=",", array=w518, 3:"%s" ("format string")) -> (spreadsheet string=w526:string)
        n173 = Enqueue Element(queue=w503, element=w501, error in (no error)=w502) -> ()  [unwired: 1 in, 3 out]
        n174 = Enqueue Element(queue=w517, element=w501, error in (no error)=w516) -> ()  [unwired: 1 in, 3 out]
        n175 = call <vilib>:"Trim Whitespace.vi"("string"=w526, "location (both)"=w527) -> ("trimmed string"=w515:string)
        "Data String" <- w515
        n176 = Concatenate Strings(w499, w443, w454, w443, w453, w443, w452, w443, w451, w443, w450, w443, w445, w443, w444, w443, w515, w443, w542, w443, w489, w443, w440, w443, w439, w443, w438, w443, w437, w443, w436, w443, w435) -> (w537:string)
        n177 = String Length(string=w537) -> (length=w541:i32)
        n178 = Number To Decimal String(number=w541, width (-)=i16 3) -> (decimal integer string=w539:string)
        n179 = Concatenate Strings(w521, w520, w538, w539, w538, w537) -> (w488:string)
        "UDP_Out" <- w488
        n180 = case shown="True" w504 {
          tunnel: w488 -> [_ w580]
          tunnel: w514 -> [_ w579]
          tunnel: w513 -> [_ w578]
          frame False {
          }
          frame True {
            n181 = Enqueue Element(queue=w579, element=w580, error in (no error)=w578) -> ()  [unwired: 1 in, 3 out]
          }
        }
        n182 = case shown="True" w486 {
          tunnel: w488 -> [w569 _]
          tunnel: w482 -> [w571 w574]
          tunnel: w481 -> [w570 w573]
          tunnel: [w566 _] -> w487
          tunnel: [w565 w572] -> w478
          frame False {
            n183 = Concatenate Strings(w569, "\r") -> (w567:string)
            n184 = Write to Text File(file (use dialog)=w571, text=w567, error in=w570) -> (refnum out=w566:refnum<file>, error out=w565:errorcluster)  [unwired: 2 out]
          }
          frame True {
            n185 = Close File(refnum=w574, error in=w573) -> (error out=w572:errorcluster)  [unwired: 1 out]
          }
        }
        n186 = node-c288() -> ()  [unwired: 1 in, 1 out]
      }
      n187 = node-c288(w40) -> ()  [unwired: 1 out]
      n188 = while {
        tunnel: w55 -> [w658]
        stop <- w659 stop-if-true
        # "Must delay to avoid 100% CPU on cRIO"
        # "Broadcast CO UDP Packet"
        n189 = call-poly <vilib>:"UDP Multicast Open.vi"("time-to-live (1)"=u16 5, "port"=u16 10000) -> ("error out"=w666:errorcluster, "connection ID"=w667:refnum<k16>)  [unwired: 8 in]
        n190 = node-c288() -> (w669:T1)  [unwired: 4 in]
        n191 = timed-loop {
          tunnel: w667 -> [w689]
          tunnel: w666 -> [w688]
          timing: w669 -> [_]
          timing-out: [_] -> w668
          shift-right: [w676] -> _
          shift-left: FALSE -> [w679]
          tunnel: [w675] -> w661
          tunnel: [w673] -> w660
          tunnel: [w671] -> w659
          tunnel: w658 -> [w670]
          stop <- w672 stop-if-true
          w671 = FALSE
          # "UDP Broadcast loop"
          n192 = node-c288() -> ()  [unwired: 1 in, 1 out]
          n193 = local read "Flight Number"() -> (w682:string)
          n194 = feedback-in #2(w682) -> ()
          n195 = feedback #2() -> (w681:string)  [unwired: 1 in]
          n196 = Not Equal?(x=w682, y=w681) -> (x != y?=w680:bool)
          n197 = String To IP(1:"239.1.4.6" ("name")) -> (0:w686:u32)
          n198 = flat-sequence {
            tunnel: w686 -> [w696]
            tunnel: w688 -> [w697]
            tunnel: w689 -> [w698]
            tunnel: [w698] -> w685
            tunnel: [w697] -> w684
            tunnel: [w696] -> w683
            tunnel: w680 -> [w695]
            tunnel: u16 50001 ("port or service name") -> [w708]
            tunnel: w685 -> [w707]
            tunnel: w684 -> [w706]
            tunnel: w683 -> [w705]
            tunnel: [w704] -> w675
            tunnel: [w703] -> w673
            tunnel: w670 -> [w701]
            frame #0 {
              n199 = feedback #3(u32 0) -> (w692:u32)
              n200 = case shown="False" w695 {
                tunnel: w692 -> [w699 _]
                tunnel: [w699 u32 0] -> w691
                frame False {
                }
                frame True {
                }
              }
              "UDP_Pack_num" <- w691
              n201 = Increment(x=w691) -> (x+1=w693:u32)
              n202 = feedback-in #3(w693) -> ()
            }
            frame #1 {
              n203 = Dequeue Element(queue=w701) -> (element=w702:string)  [unwired: 2 in, 3 out]
              n204 = UDP Write(address=w705, port or service name=w708, connection ID=w707, data in=w702, 8:w706) -> (error out=w703:errorcluster, 3:w704:refnum<k16>)  [unwired: 1 in]
            }
          }
          n205 = Select(t=FALSE, s=w679, f=TRUE) -> (s? t:f=w676:bool)
          "UDP_Out Status" <- w676
          n206 = node-c288() -> ()  [unwired: 1 in, 1 out]
          n207 = Unbundle(w673) -> ("status"=w674:bool)  [unwired: 2 out]
          n208 = Compound Arithmetic op=OR(w674, w671) -> (w672:bool)
        }
        n209 = node-c288(w668) -> ()  [unwired: 1 out]
        n210 = UDP Close(connection ID=w661, 8:w660) -> (error out=→"UDP_Out_Error Out":errorcluster)  [unwired: 1 out]
        n211 = Wait (ms)(milliseconds to wait=u32 1000) -> ()  [unwired: 1 out]
      }
      n212 = while {
        tunnel: w52 -> [w111]
        tunnel: w51 -> [w110]
        stop <- w114 stop-if-true
        # "Must delay to avoid 100% CPU on cRIO"
        # "TCP Loop writing to FISH Tank"
        n213 = TCP Open Connection(address="192.168.101.110", remote port or service name=u16 3502) -> (connection ID=w117:refnum<k5>, error out=w112:errorcluster)  [unwired: 3 in]
        n214 = case shown="No Error" w112 {
          selector: w112 -> [w122 w149]
          tunnel: w117 -> [w127 w150]
          tunnel: [w126 w150] -> w116
          tunnel: [w125 w149] -> w115
          tunnel: [w124 FALSE] -> w114
          tunnel: w111 -> [w121 _]
          tunnel: w110 -> [w120 _]
          frame No Error {
            n215 = node-c288() -> (w129:T1)  [unwired: 4 in]
            n216 = timed-loop {
              tunnel: w127 -> [w143]
              tunnel: w122 -> [w142]
              tunnel: [w141] -> w126
              tunnel: [w140] -> w125
              tunnel: [w130] -> w124
              shift-right: [w134] -> _
              shift-left: FALSE -> [w137]
              timing: w129 -> [_]
              timing-out: [_] -> w128
              tunnel: w121 -> [w133]
              tunnel: w120 -> [w132]
              stop <- w138 stop-if-true
              w130 = FALSE
              n217 = node-c288() -> ()  [unwired: 1 in, 1 out]
              n218 = Dequeue Element(queue=w133, error in (no error)=w132) -> (element=w131:string)  [unwired: 1 in, 3 out]
              n219 = Select(t=FALSE, s=w137, f=TRUE) -> (s? t:f=w134:bool)
              "TCP packet\nSend To FISH" <- w134
              n220 = TCP Write(connection ID=w143, data in=w131, error in (no error)=w142) -> (connection ID out=w141:refnum<k5>, error out=w140:errorcluster)  [unwired: 1 in, 1 out]
              n221 = Unbundle(w140) -> ("status"=w139:bool)  [unwired: 2 out]
              n222 = node-c288() -> ()  [unwired: 1 in, 1 out]
              n223 = Compound Arithmetic op=OR(w139, w130) -> (w138:bool)
            }
            n224 = node-c288(w128) -> ()  [unwired: 1 out]
          }
          frame Error {
          }
        }
        n225 = TCP Close Connection(connection ID=w116, error in (no error)=w115) -> (error out=→"FISH TCP Error Out":errorcluster)  [unwired: 1 in, 1 out]
        n226 = Wait (ms)(milliseconds to wait=u32 1000) -> ()  [unwired: 1 out]
      }
      n227 = while {
        tunnel: w50 -> [w69]
        tunnel: w49 -> [w68]
        stop <- w72 stop-if-true
        # "Must delay to avoid 100% CPU on cRIO"
        # "TCP Loop writing to SEPTIC Tank"
        n228 = TCP Open Connection(address="192.168.101.108", remote port or service name=u16 3502) -> (connection ID=w75:refnum<k5>, error out=w70:errorcluster)  [unwired: 3 in]
        n229 = case shown="No Error" w70 {
          selector: w70 -> [w80 w107]
          tunnel: w75 -> [w85 w108]
          tunnel: [w84 w108] -> w74
          tunnel: [w83 w107] -> w73
          tunnel: [w82 FALSE] -> w72
          tunnel: w69 -> [w79 _]
          tunnel: w68 -> [w78 _]
          frame No Error {
            n230 = node-c288() -> (w87:T1)  [unwired: 4 in]
            n231 = timed-loop {
              tunnel: w85 -> [w101]
              tunnel: w80 -> [w100]
              tunnel: [w99] -> w84
              tunnel: [w98] -> w83
              tunnel: [w88] -> w82
              shift-right: [w92] -> _
              shift-left: FALSE -> [w95]
              timing: w87 -> [_]
              timing-out: [_] -> w86
              tunnel: w79 -> [w91]
              tunnel: w78 -> [w90]
              stop <- w96 stop-if-true
              w88 = FALSE
              n232 = node-c288() -> ()  [unwired: 1 in, 1 out]
              n233 = Dequeue Element(queue=w91, error in (no error)=w90) -> (element=w89:string)  [unwired: 1 in, 3 out]
              n234 = Select(t=FALSE, s=w95, f=TRUE) -> (s? t:f=w92:bool)
              "TCP packet\nSend To SEPTIC" <- w92
              n235 = TCP Write(connection ID=w101, data in=w89, error in (no error)=w100) -> (connection ID out=w99:refnum<k5>, error out=w98:errorcluster)  [unwired: 1 in, 1 out]
              n236 = Unbundle(w98) -> ("status"=w97:bool)  [unwired: 2 out]
              n237 = node-c288() -> ()  [unwired: 1 in, 1 out]
              n238 = Compound Arithmetic op=OR(w97, w88) -> (w96:bool)
            }
            n239 = node-c288(w86) -> ()  [unwired: 1 out]
          }
          frame Error {
          }
        }
        n240 = TCP Close Connection(connection ID=w74, error in (no error)=w73) -> (error out=→"SEPTIC TCP Error Out":errorcluster)  [unwired: 1 in, 1 out]
        n241 = Wait (ms)(milliseconds to wait=u32 1000) -> ()  [unwired: 1 out]
      }
      n242 = while {
        stop <- FALSE stop-if-true
        n243 = node-c288() -> (w371:T1)  [unwired: 4 in]
        n244 = Create Network Stream Reader Endpoint(7:10 ("reader buffer size"), 9:T4 {"Message"="", "Message Data"=variant} ("Message Cluster"), 11:"/command/reader/CO" ("reader url")) -> (0:w377:errorcluster, 3:w378:refnum<k21>)  [unwired: 4 in]
        n245 = timed-loop "Host->Target Command Reader" {
          shift-right: [w388] -> w375
          shift-left: w377 -> [w391]
          shift-right: [w389] -> w374
          shift-left: w378 -> [w390]
          tunnel: [TRUE] -> _
          timing: w371 -> [_]
          timing-out: [_] -> w370
          stop <- w382 stop-if-true
          # "Receive Commands from Host VI"
          n246 = node-c288() -> ()  [unwired: 1 in, 1 out]
          n247 = shared-variable-read(w390, w391) -> (w389:refnum<k21>, w384:errorcluster, w386:bool, w387:T4)  [unwired: 1 in]
          n248 = Or(x=w386, y=w384) -> (x .or. y?=w385:bool)
          n249 = case shown="False" w385 {
            selector: w385 -> [_ w428]
            tunnel: w384 -> [w399 w429]
            tunnel: [w398 w429] -> w388
            tunnel: w387 -> [w397 _]
            tunnel: [w394 w428] -> w382
            frame False {
              n250 = Unbundle By Name(w397) -> ("Message"=w396:string, "Message Data"=w395:variant)
              n251 = case shown="\"UDP Time Offset\"" w396 {
                tunnel: w399 -> [w403 w408 w410 w416 w422 w427]
                tunnel: [w400 w405 w410 w415 w421 w426] -> w398
                tunnel: w395 -> [w404 w409 _ w414 w420 w425]
                tunnel: [_ _ TRUE _ _ _] -> w394
                frame "Stop File Write" {
                  n252 = Variant To Data(error in=w403, type=FALSE, Variant=w404) -> (data=→"Stop File Write":bool, error out=w400:errorcluster)
                }
                frame "Flight Number" {
                  n253 = Variant To Data(error in=w408, type="", Variant=w409) -> (data=→"Flight Number":string, error out=w405:errorcluster)
                }
                frame "Stop", Default {
                }
                frame "CO CAL" {
                  n254 = Variant To Data(error in=w416, type=FALSE, Variant=w414) -> (data=→"CO CAL":bool, error out=w415:errorcluster)
                }
                frame "CO Vacuum" {
                  n255 = Variant To Data(error in=w422, type=FALSE, Variant=w420) -> (data=w417:bool, error out=w421:errorcluster)
                  "CO Vacuum" <- w417
                  n256 = Boolean To (0,1)(Boolean=w417) -> (0, 1=→"CO Vacuum?":i16)
                  n257 = shared-variable "NI-cRIO9022-019C2C95\\Mod6\\DO5"(w417) -> ()  [unwired: 1 in, 1 out]
                }
                frame "UDP Time Offset" {
                  n258 = Variant To Data(error in=w427, type=0, Variant=w425) -> (data=→"UDP Time Stamp Offset":i32, error out=w426:errorcluster)
                }
              }
            }
            frame True {
            }
          }
          n259 = node-c288() -> ()  [unwired: 1 in, 1 out]
        }
        n260 = node-c288(w370) -> ()  [unwired: 1 out]
        n261 = Destroy Stream Endpoint(8:w375, 11:w374) -> (0:→"error out":errorcluster)
        n262 = Wait (ms)(milliseconds to wait=u32 1000) -> ()  [unwired: 1 out]
      }
      n263 = node-c288(w38) -> ()  [unwired: 1 out]
    }
    frame Error {
    }
  }
  n264 = disable-structure shown="Enabled" {
    frame Disabled {
      n265 = while {
        stop <- FALSE stop-if-true
        # "Must delay to avoid 100% CPU on cRIO"
        # "CO Control Data Loop"
        n266 = call <vilib>:"TCP Listen.vi"("port"=u16 1002) -> ("error out"=w719:errorcluster, "connection ID"=w720:refnum<k5>)  [unwired: 6 in, 3 out]
        n267 = node-c288() -> (w723:T1)  [unwired: 4 in]
        n268 = timed-loop {
          timing: w723 -> [_]
          timing-out: [_] -> w722
          tunnel: w720 -> [w740]
          tunnel: w719 -> [w739]
          tunnel: [w729] -> w718
          tunnel: [w728] -> w717
          stop <- w728 stop-if-true
          n269 = node-c288() -> ()  [unwired: 1 in, 1 out]
          n270 = TCP Read(connection ID=w740, bytes to read=4, error in (no error)=w739) -> (connection ID out=w737:refnum<k5>, data out=w734:string, error out=w736:errorcluster)  [unwired: 2 in]
          n271 = Type Cast(type=0, x=w734) -> (*(type *) &x=w733:i32)
          n272 = TCP Read(connection ID=w737, bytes to read=w733, error in (no error)=w736) -> (connection ID out=w729:refnum<k5>, data out=w730:string, error out=w728:errorcluster)  [unwired: 2 in]
          "Control data out" <- w730
          n273 = Spreadsheet String To Array(delimiter (Tab)=",", format string="%b", spreadsheet string=w730, array type (2D Dbl)=i32[] []) -> (array=w727:i32[])
          "Control data" <- w727
          n274 = Index Array(array=w727) -> (element #2=w725:i32)  [unwired: 2 in, 1 out]
          n275 = Not Equal To 0?(x=w725) -> (x != 0?=w724:bool)
          n276 = shared-variable "NI-cRIO9022-019C2C95\\Mod6\\DO5"(w724) -> ()  [unwired: 1 in, 1 out]
          n277 = node-c288() -> ()  [unwired: 1 in, 1 out]
        }
        n278 = Wait (ms)(milliseconds to wait=u32 1000) -> ()  [unwired: 1 out]
        n279 = node-c288(w722) -> ()  [unwired: 1 out]
        n280 = TCP Close Connection(connection ID=w718, error in (no error)=w717) -> ()  [unwired: 1 in, 2 out]
      }
    }
    frame Enabled {
    }
  }
  n281 = VISA Close(VISA resource name=w14, error in (no error)=w15) -> (error out=→"Serial VISA error":errorcluster)
